vi "write data.vi"(8 "error in (no error)":errorcluster, 10 "data":string, 11 "Device in":T1) -> (0 "error out":errorcluster, 3 "Device out":T1)   [LabVIEW 2015]
uses:
  typedefs/device.ctl
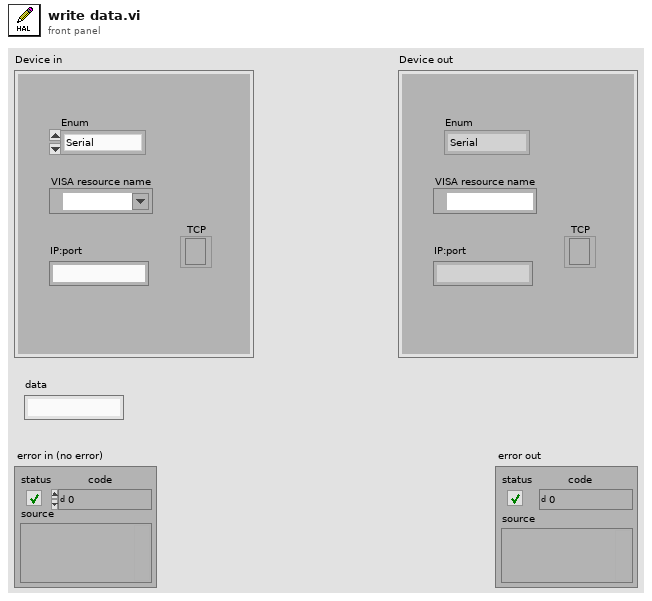
[diagram p1: front panel]
types:
  T1 = typedef "device.ctl" = cluster{"Enum":enum16{"Serial", "TCP/IP", "Mock"}, "IP:port":string, "VISA resource name":refnum<visa-resource-name>, "TCP":refnum<k5>}
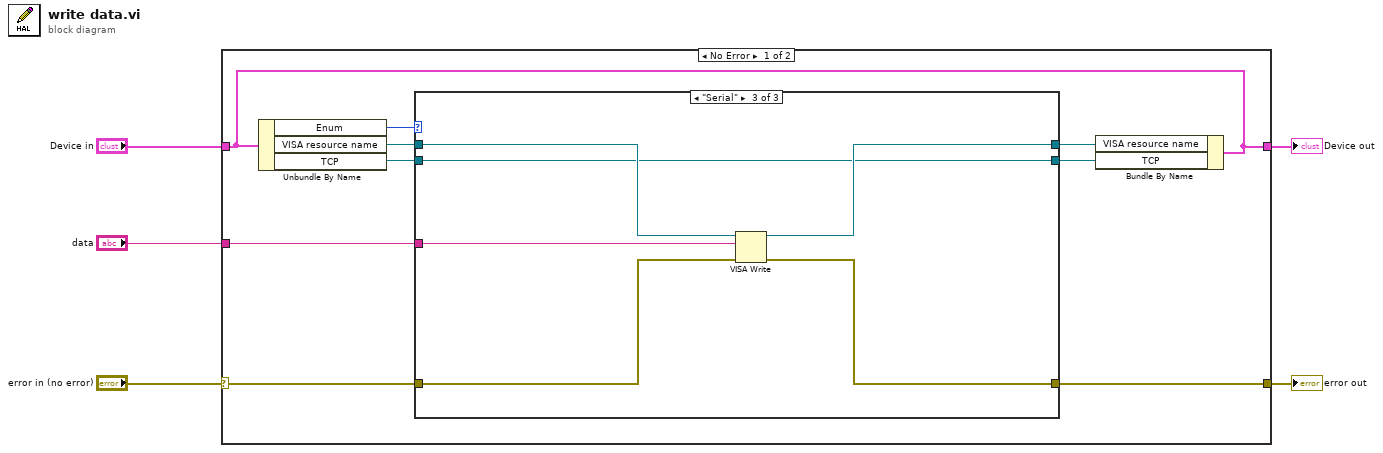
[diagram p0: block diagram]
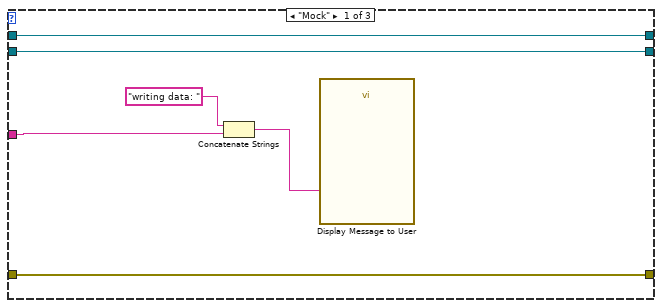
[diagram p2: hidden frame]
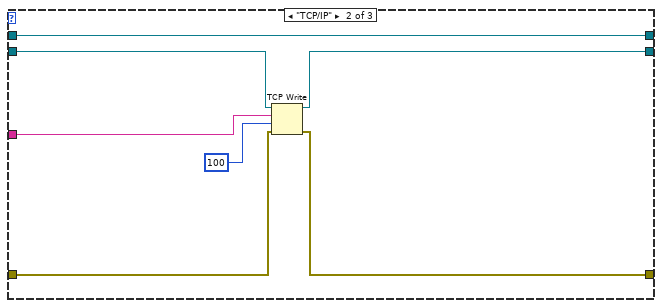
[diagram p3: hidden frame]
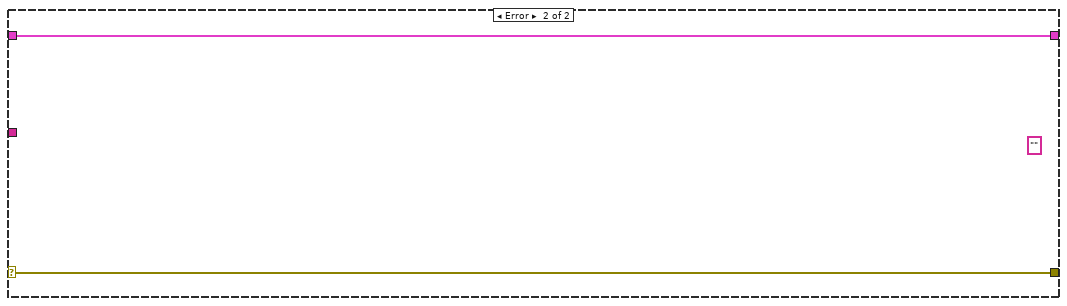
[diagram p4: hidden frame]
diagram:
  n1 = case shown="No Error" "error in (no error)" {
    selector: "error in (no error)" -> [w14 w34]
    tunnel: [w9 w35] -> w4
    tunnel: "Device in" -> [w9 w35]
    tunnel: [w13 w34] -> w2
    tunnel: "data" -> [w8 _]
    frame No Error {
      n2 = Unbundle By Name(w9) -> ("Enum"=w11:enum16{"Serial", "TCP/IP", "Mock"}, "VISA resource name"=w12:refnum<visa-resource-name>, "TCP"=w7:refnum<k5>)
      n3 = case shown="\"Serial\"" w11 {
        tunnel: w12 -> [w20 w27 w32]
        tunnel: w14 -> [w19 w23 w33]
        tunnel: [w19 w22 w29] -> w13
        tunnel: [w20 w27 w30] -> w10
        tunnel: w8 -> [w17 w24 w31]
        tunnel: w7 -> [w15 w26 w28]
        tunnel: [w15 w25 w28] -> w6
        frame "Mock" {
          n4 = Concatenate Strings("writing data: ", w17) -> (w16:string)
          n5 = call "Display Message to User"("Message"=w16) -> ()  [unwired: 9 in, 2 out]
        }
        frame "TCP/IP" {
          n6 = TCP Write(connection ID=w26, data in=w24, error in (no error)=w23, 9:100 ("timeout ms (25000)")) -> (connection ID out=w25:refnum<k5>, error out=w22:errorcluster)  [unwired: 1 out]
        }
        frame "Serial" {
          n7 = VISA Write(VISA resource name=w32, write buffer=w31, error in (no error)=w33) -> (VISA resource name out=w30:refnum<visa-resource-name>, error out=w29:errorcluster)  [unwired: 1 out]
        }
      }
      n8 = Bundle By Name(cluster=w9, "VISA resource name"=w10, "TCP"=w6) -> ()  [unwired: 1 out]
    }
    frame Error {
      (unwired) "" ("read buffer")
    }
  }
  "error out" <- w2
  "Device out" <- w4
